vi "test Should Return Call Parameters If Read Multiple Times.vi"(8 "error in (no error)":errorcluster, 11 "TestCase in":refnum<class "Store and Return Parameters.lvclass">) -> (0 "error out":errorcluster, 3 "TestCase out":refnum<class "Store and Return Parameters.lvclass">)   [LabVIEW 2013, in "Store and Return Parameters.lvclass"]
uses:
  Store and Return Parameters.lvclass
  Core Classes/LabSpy/LabSpy.lvclass
  <vilib>/addons/_JKI Toolkits/VI Tester/TestCase.llb/TestCase.lvclass
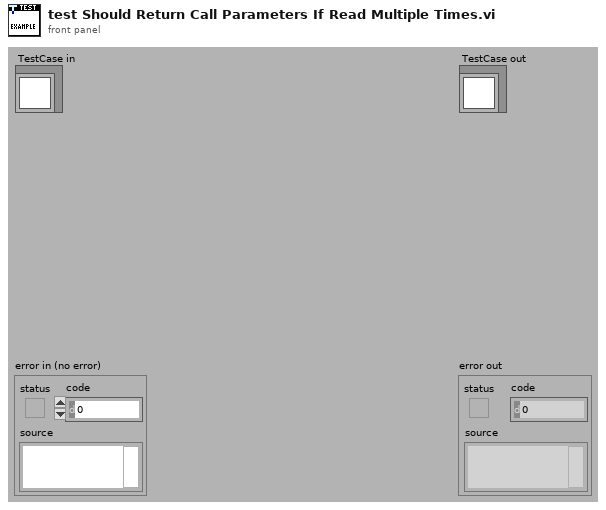
[diagram p1: front panel]
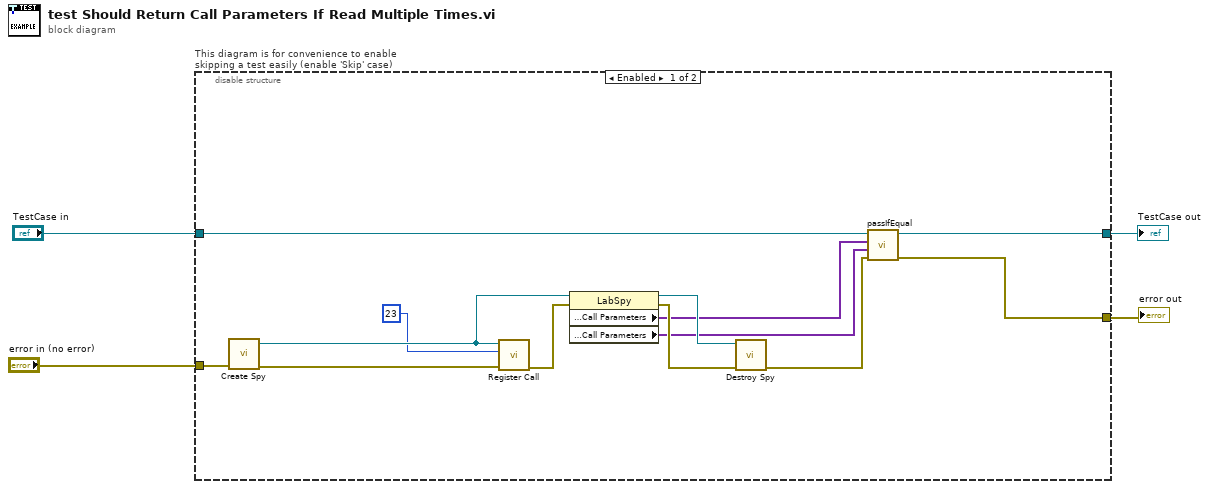
[diagram p0: block diagram]
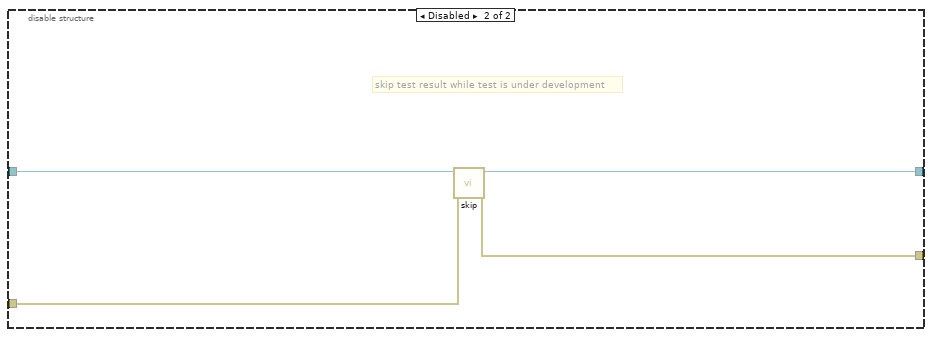
[diagram p2: hidden frame]
diagram:
  n1 = disable-structure "This diagram is for convenience to enable skipping a test easily (enable 'Skip' case)" shown="Enabled" {
    disable-tunnel: "TestCase in" -> [w11 w21]
    disable-tunnel: [w8 w19] -> w1
    disable-tunnel: [w7 w20] -> w3
    disable-tunnel: "error in (no error)" -> [w17 w18]
    frame Enabled {
      n2 = call "Create Spy.vi"("error in (no error)"=w17) -> ("error out"=w16:errorcluster, "LabSpy Out"=w15:refnum<data-value>)  [unwired: 9 in]
      n3 = call "Register Call.vi"("error in (no error)"=w16, "Parameters"=23, "LabSpy"=w15) -> ("error out"=w14:errorcluster)  [unwired: 7 in, 1 out]
      n4 = property class="LabSpy"(reference=w15, error in=w14) -> (reference out=w12:refnum<data-value>, error out=w13:errorcluster, "Parameter Readings:Call Parameters"=w5:variant[], "Parameter Readings:Call Parameters"=w6:variant[])
      n5 = call "Destroy Spy.vi"("error in (no error)"=w13, "LabSpy"=w12) -> ("error out"=w10:errorcluster)  [unwired: 9 in]
      n6 = call-dynamic "passIfEqual.vi"("error in (no error)"=w10, "y"=w6, "x"=w5, "TestCase in"=w11) -> ("error out"=w7:errorcluster, "TestCase out"=w8:refnum<class "Store and Return Parameters.lvclass">)  [unwired: 6 in]
    }
    frame Disabled {
      # "skip test result while test is under development"
      n7 = call <vilib>:"skip.vi"("error in (no error)"=w18, "TestCase in"=w21) -> ("error out"=w20:errorcluster, "TestCase out"=w19:refnum<class "Store and Return Parameters.lvclass">)  [unwired: 8 in]
    }
  }
  "error out" <- w3
  "TestCase out" <- w1
